vi "ROI group interface-Find POI within group boundaries 2.vi"(8 "error in (no error)":errorcluster, 9 "X-Y coordinates array of POI":dbl[][](array[numeric]), 10 "ROI Descriptor Out":T2 {"Contours"."Type" items=["No Selection", "Point", "Line", "Rectangle", "Oval", "Polygon", "Freehand Region", "Annulus", "Unused2", "Unused3", "Broken Line", "Freehand Line", "Rotated Rectangle"]}, 11 "Image ref in":T1) -> (0 "error out":errorcluster, 1 "# of POI in group":i32, 2 "ROI to be grouped":i32[](array[numeric]), 3 "Image ref shift out":T1)   [LabVIEW 2020]
uses:
  <vilib>/vision/Image Controls.llb/IMAQ Image.ctl
  <vilib>/vision/NI_Vision_Development_Module.lvlib
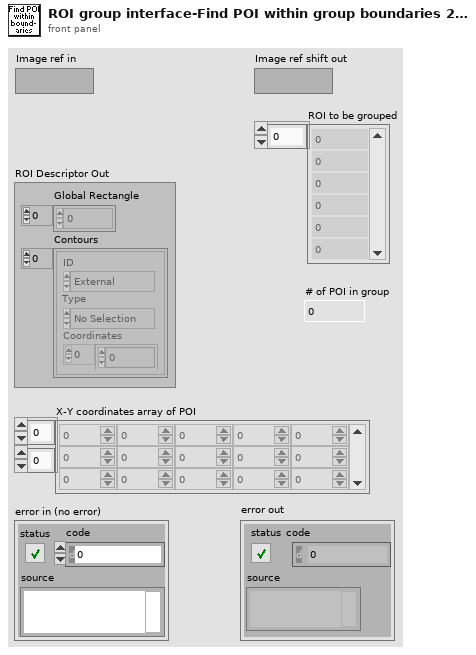
[diagram p1: front panel]
types:
  T1 = typedef "IMAQ Image.ctl" = refnum<image>
  T2 = typedef "ROI Descriptor" = cluster{"Global Rectangle":i32[], "Contours":cluster{"ID":enum32{"External", "Internal"}, "Type":u32, "Coordinates":i32[]}[]}
  T3 = typedef "IMAQ Point" = cluster{"X":sgl, "Y":sgl}
  T4 = typedef "Image Type" = u32
  T5 = cluster{"histogram":u32[], "Minimal Value":sgl, "Maximal Value":sgl, "Starting Value":sgl, "Interval Width":sgl, "Mean Value":sgl, "Standard  Variation":sgl, "Area (pixels)":i32}
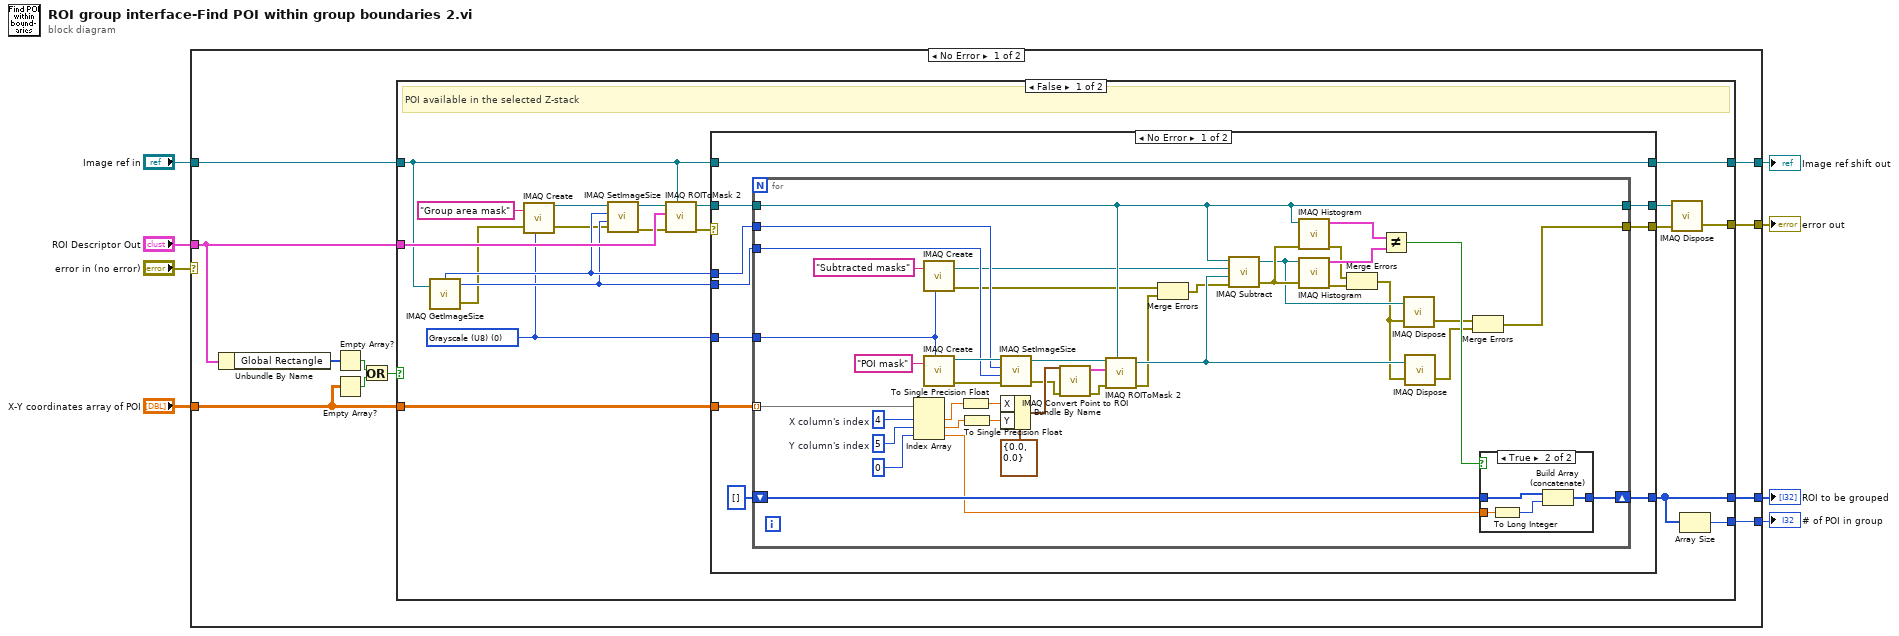
[diagram p0: block diagram]
diagram:
  n1 = case shown="No Error" "error in (no error)" {
    selector: "error in (no error)" -> [_ w101]
    tunnel: [w19 _] -> w8
    tunnel: [w18 _] -> w7
    tunnel: "ROI Descriptor Out" -> [w13 _]
    tunnel: "Image ref in" -> [w17 w100]
    tunnel: [w16 w101] -> w5
    tunnel: "X-Y coordinates array of POI" -> [w15 _]
    tunnel: [w14 w100] -> w2
    frame No Error {
      n2 = Unbundle By Name(w13) -> ("Global Rectangle"=w12:i32[])
      n3 = Empty Array?(array=w12) -> (empty?=w11:bool)
      n4 = Empty Array?(array=w15) -> (empty?=w10:bool)
      n5 = Or(x=w11, y=w10) -> (x .or. y?=w9:bool)
      n6 = case shown="False" w9 {
        tunnel: [w35 _] -> w19
        tunnel: [w34 _] -> w18
        tunnel: w13 -> [w33 _]
        tunnel: w17 -> [w21 w99]
        tunnel: [w29 _] -> w16
        tunnel: w15 -> [w28 _]
        tunnel: [w27 w99] -> w14
        frame False {
          w20 = T4 0 items=["Grayscale (U8)", "Grayscale (I16)", "Grayscale (SGL)", "Complex (CSG)", "RGB (U32)", "HSL (U32)", "RGB (U64)", "Grayscale (U16)"] ("Image Type")
          # "POI available in the selected Z-stack"
          n7 = call "IMAQ GetImageSize"("Image"=w21) -> ("Y Resolution"=w25:i32, "X Resolution"=w26:i32, "error out"=w23:errorcluster)  [unwired: 3 in]
          n8 = call "IMAQ Create"("Image Name"="Group area mask" ("string"), "Image Type"=w20, "error in (no error)"=w23) -> ("New Image"=w38:T1, "error out"=w24:errorcluster)  [unwired: 2 in]
          n9 = call "IMAQ SetImageSize"("error in (no error)"=w24, "Y Resolution"=w25, "X Resolution"=w26, "Image"=w38) -> ("error out"=w32:errorcluster, "Image Out"=w22:T1)  [unwired: 1 in]
          n10 = call "IMAQ ROIToMask 2"("Image Model"=w21, "error in (no error)"=w32, "ROI Descriptor"=w33, "Image"=w22) -> ("error out"=w31:errorcluster, "Image Out"=w36:T1)  [unwired: 5 in, 1 out]
          n11 = case shown="No Error" w31 {
            selector: w31 -> [_ w98]
            tunnel: [w49 w97] -> w39
            tunnel: w36 -> [w48 w97]
            tunnel: [w47 _] -> w34
            tunnel: w28 -> [w45 _]
            tunnel: w21 -> [w43 w96]
            tunnel: [w46 w98] -> w30
            tunnel: [w43 w96] -> w27
            tunnel: w26 -> [w42 _]
            tunnel: w25 -> [w41 _]
            tunnel: w20 -> [w40 _]
            frame No Error {
              n12 = for {
                tunnel: w48 -> [w63]
                tunnel: w45 -> [w86] mode=indexing
                shift-right: [w75] -> w47
                shift-left: i32[] [] -> [w74]
                tunnel: [w63] -> w49
                tunnel: [w70] -> w46
                tunnel: w42 -> [w68]
                tunnel: w41 -> [w67]
                tunnel: w40 -> [w66]
                w51 = 5  # Y column's index
                w50 = 4  # X column's index
                n13 = Index Array(array=w86, index #1=w50, index #2=w51, index #3=0 ("index")) -> (element #1=w85:dbl, element #2=w84:dbl, element #3=w53:dbl)
                n14 = call "IMAQ Create"("Image Name"="Subtracted masks" ("string"), "Image Type"=w66) -> ("New Image"=w60:T1, "error out"=w59:errorcluster)  [unwired: 3 in]
                n15 = call "IMAQ Create"("Image Name"="POI mask" ("string"), "Image Type"=w66) -> ("New Image"=w81:T1, "error out"=w73:errorcluster)  [unwired: 3 in]
                n16 = To Single Precision Float(number=w85) -> (single precision float=w62:sgl)
                n17 = To Single Precision Float(number=w84) -> (single precision float=w61:sgl)
                n18 = call "IMAQ SetImageSize"("error in (no error)"=w73, "Y Resolution"=w67, "X Resolution"=w68, "Image"=w81) -> ("error out"=w55:errorcluster, "Image Out"=w65:T1)  [unwired: 1 in]
                n19 = Bundle By Name(cluster=T3 {"X"=0.0, "Y"=0.0} ("Point"), "X"=w62, "Y"=w61) -> (w83:T3)
                n20 = call "IMAQ Convert Point to ROI"("error in (no error)"=w55, "Point"=w83) -> ("error out"=w54:errorcluster, "ROI Descriptor"=w90:T2)  [unwired: 7 in]
                n21 = call "IMAQ ROIToMask 2"("Image Model"=w63, "error in (no error)"=w54, "ROI Descriptor"=w90, "Image"=w65) -> ("error out"=w58:errorcluster, "Image Out"=w69:T1)  [unwired: 5 in, 1 out]
                n22 = Merge Errors(w59, w58) -> (w57:errorcluster)
                n23 = call "IMAQ Subtract"("Image Src A"=w63, "Image Dst"=w60, "Image Src B"=w69, "error in (no error)"=w57) -> ("Image Dst Out"=w64:T1, "error out"=w79:errorcluster)  [unwired: 3 in]
                n24 = call "IMAQ Histogram"("error in (no error)"=w79, "Image"=w63) -> ("error out"=w78:errorcluster, "Histogram Report"=w89:T5)  [unwired: 8 in]
                n25 = call "IMAQ Histogram"("error in (no error)"=w79, "Image"=w64) -> ("error out"=w77:errorcluster, "Histogram Report"=w88:T5)  [unwired: 8 in]
                n26 = Merge Errors(w78, w77) -> (w56:errorcluster)
                n27 = Not Equal?(x=w89, y=w88) -> (x != y?=w76:bool)
                n28 = call "IMAQ Dispose"("Image"=w64, "error in (no error)"=w56) -> ("error out"=w72:errorcluster)  [unwired: 4 in]
                n29 = call "IMAQ Dispose"("Image"=w69, "error in (no error)"=w56) -> ("error out"=w71:errorcluster)  [unwired: 4 in]
                n30 = Merge Errors(w72, w71) -> (w70:errorcluster)
                n31 = case shown="True" w76 {
                  tunnel: [w91 w95] -> w75
                  tunnel: w74 -> [w91 w94]
                  tunnel: w53 -> [_ w93]
                  frame False {
                  }
                  frame True {
                    n32 = To Long Integer(number=w93) -> (32bit integer=w92:i32)
                    n33 = Build Array (concatenate)(w94, w92) -> (w95:i32[])
                  }
                }
              }
            }
            frame Error {
            }
          }
          n34 = call "IMAQ Dispose"("Image"=w39, "error in (no error)"=w30) -> ("error out"=w29:errorcluster)  [unwired: 4 in]
          n35 = Array Size(array=w34) -> (size(s)=w35:i32)
        }
        frame True {
          # "No POI available in the selected Z-stack OR no POI selected by drawing a circle around them"
        }
      }
    }
    frame Error {
    }
  }
  "ROI to be grouped" <- w7
  "# of POI in group" <- w8
  "error out" <- w5
  "Image ref shift out" <- w2
